vi "analogWaveforms.vi"() -> ()   [LabVIEW 2009, in "run.lvlib"]
doc: "I. Description:\nThis example demonstrates how to continuously output a waveform using an internal sample clock and a digital start trigger.\n\nII. Instructions for Running:\n1. Select the Physical Channel to correspond to where your signal is output on the DAQ device.\n2. Enter the Minimum and Maximum Voltage Ranges.\n3. Specify the Desired Frequency of the output Waveform\n4. Select the Digital Trigger Source.\n5. Specify the desired Trigger Edge.\n6. Enter the Waveform Information. See the documentation of the Waveform Buffer Generation SubVI for information on each parameter.\n\nIII. Block Diagram Steps:\n1. Create an Analog Output Voltage Task\n2.Call the DAQmx Timing (Use Waveform) VI which sets the sample clock rate based on the input waveform parameters, and set the sample mode to Continuous.\n3. Define the Triggering parameters: Source and Edge\n4. Write the waveform to the output buffer.\n5. Call the Start VI.\n6. Loop continuously until the user presses the Stop button. Check for errors every 100 ms using the Is Task Done? VI\n7. Call the Clear Task VI to clear the Task.\n8. Use the popup dialog box to display an error or warning if any.\n\nIV. I/O Connections Overview:\nMake sure your signal output terminal matches the Physical Channel I/O Control. Also, make sure your digital trigger terminal matches the Trigger Source Control. For further connection information, refer to your hardware reference manual."
uses:
  <vilib>/Utility/error.llb/DialogType.ctl
  <vilib>/DAQmx/write.llb/DAQmx Write (Analog 1D Wfm NChan NSamp).vi
  <vilib>/DAQmx/configure/timing.llb/DAQmx Timing (Use Waveform).vi
  <vilib>/DAQmx/create/channels.llb/DAQmx Create Channel (AO-Voltage-Basic).vi
  Hal/testing/run.lvlib
panel:
  in  "Cycles per Buffer":i32=15
  in  "Waveform Type":T1(ring)
  in  "Amplitude":dbl=2.0 format="%0.2p"
  in  "Samples per Buffer":dbl=750.0
  in  "Desired Frequency":dbl=1000.0 format="%.2f"
  out "Output Waveform":waveform(dbl)[](graph)
  in  "Physical Channels":tag="Dev1/ao0:1"
  in  "Minimum Value":dbl=-10.0 format="%0.2f"
  in  "Maximum Value":dbl=10.0 format="%0.2f"
  in  "stop":bool
  # "For instructions, select Help>>Show Context Help"
  # "Channel Parameters"
  # "Waveform Information"
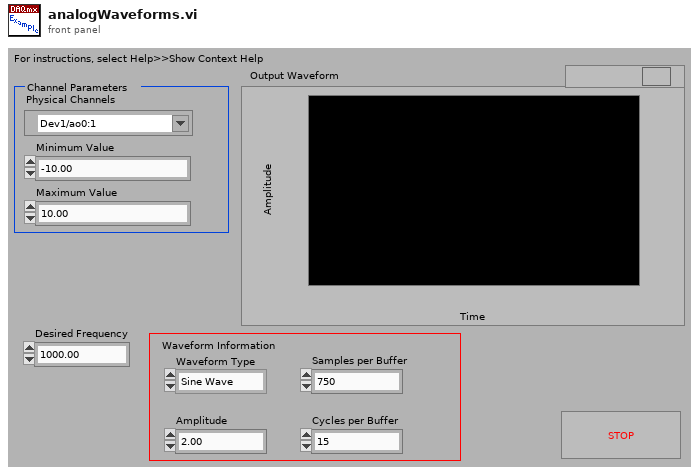
[diagram p1: front panel]
types:
  T1 = enum16{"Sine Wave", "Triangle Wave", "Square Wave", "Sawtooth Wave"}
  T2 = typedef "DialogType.ctl" = u16
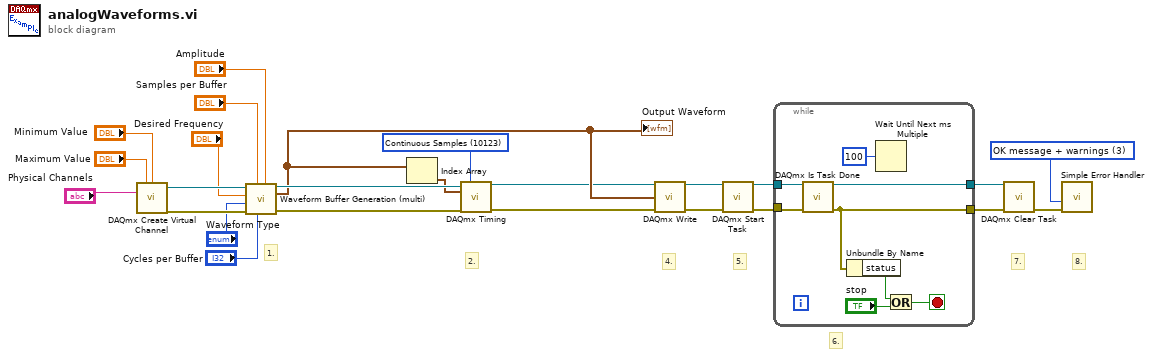
[diagram p0: block diagram]
diagram:
  w17 = T2 3 items=["no dialog", "OK message", "continue or stop message", "OK message + warnings", "continue/stop + warnings"] ("type of dialog (OK msg:1)")
  w24 = 10123 items=["Finite Samples"=10178, "Continuous Samples"=10123] ("sample mode")
  # "8."
  # "6."
  # "7."
  # "5."
  # "4."
  # "2."
  # "1."
  n1 = call-poly <vilib>:"DAQmx Create Virtual Channel.vi"("maximum value"="Maximum Value", "minimum value"="Minimum Value", "physical channels"="Physical Channels") -> ("task out"=w11:refnum<k21>, "error out"=w13:errorcluster)  [unwired: 11 in]
  n2 = call "Waveform Buffer Generation (multi).vi"("Amplitude"="Amplitude", "Cycles per Buffer"="Cycles per Buffer", "Samples per Buffer"="Samples per Buffer", "error in (no error)"=w13, "Waveform Type"="Waveform Type", "Desired Frequency"="Desired Frequency", "task/channels in"=w11) -> ("error out"=w12:errorcluster, "Waveform"=w4:waveform(dbl)[], "task out"=w5:refnum<k21>)  [unwired: 2 out]
  "Output Waveform" <- w4
  n3 = Index Array(array=w4) -> (element=w3:waveform(dbl))  [unwired: 1 in]
  n4 = call-poly <vilib>:"DAQmx Timing.vi"("task/channels in"=w5, "sample mode"=w24, "waveform"=w3, "error in"=w12) -> ("task out"=w2:refnum<k21>, "error out"=w1:errorcluster)  [unwired: 10 in]
  n5 = call-poly <vilib>:"DAQmx Write.vi"("task/channels in"=w2, "data"=w4, "error in"=w1) -> ("task out"=w21:refnum<k21>, "error out"=w20:errorcluster)  [unwired: 10 in, 1 out]
  n6 = call <vilib>:"DAQmx Start Task.vi"("task/channels in"=w21, "error in"=w20) -> ("task out"=w25:refnum<k21>, "error out"=w19:errorcluster)  [unwired: 12 in]
  n7 = while {
    tunnel: w25 -> [w29]
    tunnel: [w26] -> w15
    tunnel: w19 -> [w28]
    tunnel: [w27] -> w14
    stop <- w33 stop-if-true
    n8 = call <vilib>:"DAQmx Is Task Done.vi"("task/channels in"=w29, "error in"=w28) -> ("task out"=w26:refnum<k21>, "error out"=w27:errorcluster)  [unwired: 11 in, 1 out]
    n9 = Unbundle By Name(w27) -> ("status"=w31:bool)
    n10 = Wait Until Next ms Multiple(millisecond multiple=u32 100) -> ()  [unwired: 1 out]
    n11 = Or(x=w31, y="stop") -> (x .or. y?=w33:bool)
  }
  n12 = call <vilib>:"DAQmx Clear Task.vi"("task in"=w15, "error in"=w14) -> ("error out"=w16:errorcluster)  [unwired: 13 in]
  n13 = call <vilib>:"Simple Error Handler.vi"("type of dialog (OK msg:1)"=w17, "error in (no error)"=w16) -> ()  [unwired: 3 in, 5 out]
